vi "Write Value.vi"(8 "error in (no error)":errorcluster, 10 "Abs_Value.lvclass":refnum<class "Abs_Value.lvclass">, 11 "Assign abs_Value in":refnum<class "Assign abs_Value.lvclass">) -> (0 "error out":errorcluster, 3 "Assign abs_Value out":refnum<class "Assign abs_Value.lvclass">)   [LabVIEW 2021, in "BT.lvlib" / "Assign abs_Value.lvclass"]
uses:
  Assign abs_Value.lvclass
  <vilib>/TSA/Abstract Data Classes/Abs_Types/Value/Abs_Value.lvclass
  Assign abs_Value.lvclass/Assign abs_Value.ctl
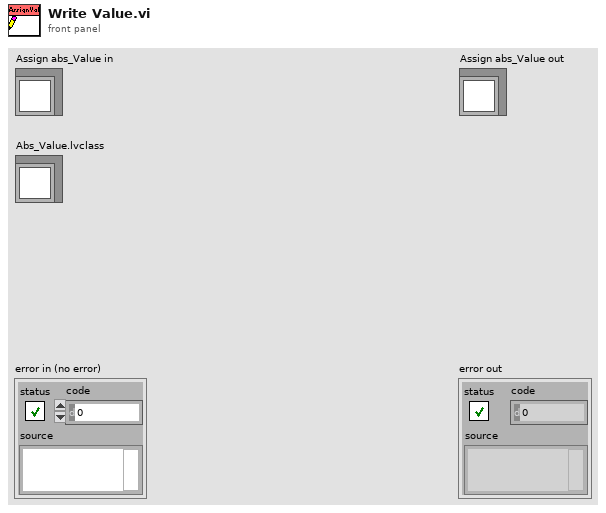
[diagram p1: front panel]
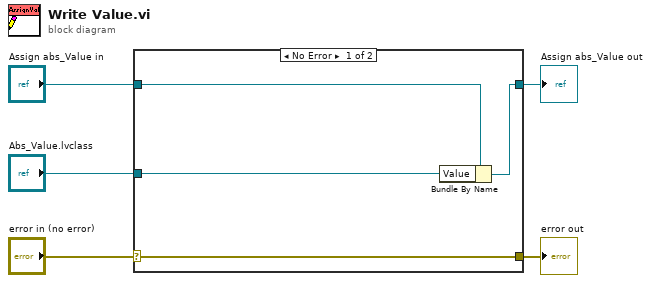
[diagram p0: block diagram]
diagram:
  n1 = case shown="No Error" "error in (no error)" {
    selector: "error in (no error)" -> [w9 w10]
    tunnel: [w9 w10] -> w4
    tunnel: [w7 w11] -> w2
    tunnel: "Assign abs_Value in" -> [w8 w11]
    tunnel: "Abs_Value.lvclass" -> [w6 _]
    frame No Error {
      n2 = Bundle By Name(cluster=w8, "Value"=w6) -> (w7:refnum<class "Assign abs_Value.lvclass">)
    }
    frame Error {
    }
  }
  "error out" <- w4
  "Assign abs_Value out" <- w2
